vi "factorial.vi"(1 "n":u32) -> (0 "factorial":u32)   [LabVIEW 2019]
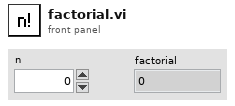
[diagram p1: front panel]
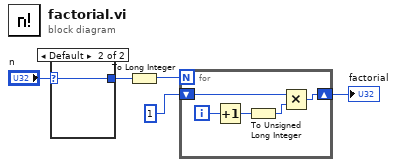
[diagram p0: block diagram]
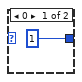
[diagram p2: hidden frame]
diagram:
  n1 = case shown="Default" "n" {
    selector: "n" -> [_ w7]
    tunnel: [u32 1 ("n") w7] -> w3
    frame 0 {
    }
    frame Default {
    }
  }
  n2 = To Long Integer(number=w3) -> (32bit integer=w5:i32)
  n3 = for {
    N: w5 -> [_]
    shift-right: [w8] -> w1
    shift-left: u32 1 ("n") -> [w11]
    i -> [w12]
    n4 = Increment(x=w12) -> (x+1=w10:i32)
    n5 = To Unsigned Long Integer(number=w10) -> (unsigned 32bit integer=w9:u32)
    n6 = Multiply(x=w11, y=w9) -> (x*y=w8:u32)
  }
  "factorial" <- w1
